vi "报警信息.vi"(11 "报警簇":bool[](array[boolean])) -> (2 "系统报警信息":string, 3 "采配水报警信息":string)   [LabVIEW 2016, in "PLC.lvlib"]
uses:
  PLC.lvlib
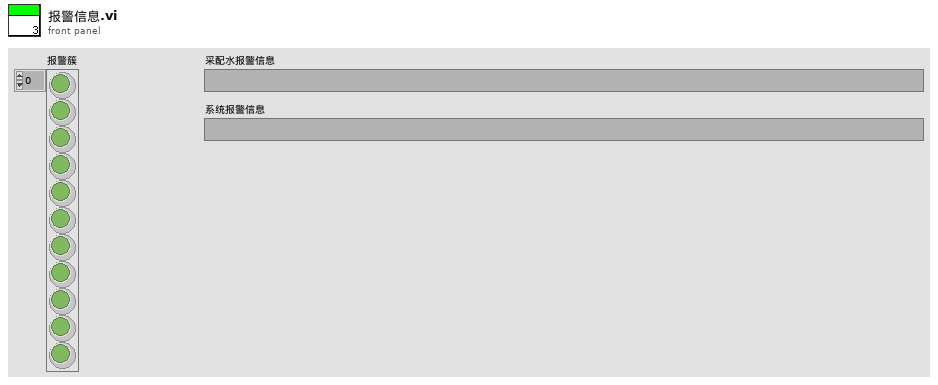
[diagram p1: front panel]
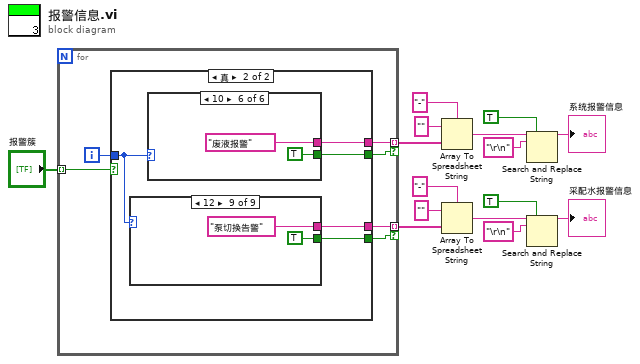
[diagram p0: block diagram]
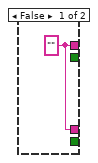
[diagram p2: hidden frame]
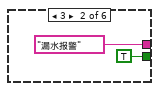
[diagram p4: hidden frame]
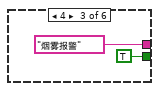
[diagram p5: hidden frame]
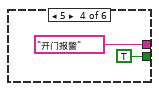
[diagram p6: hidden frame]
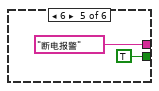
[diagram p7: hidden frame]
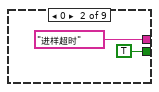
[diagram p9: hidden frame]
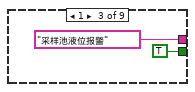
[diagram p10: hidden frame]
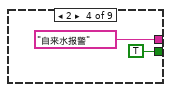
[diagram p11: hidden frame]
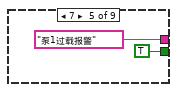
[diagram p12: hidden frame]
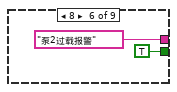
[diagram p13: hidden frame]
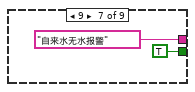
[diagram p14: hidden frame]
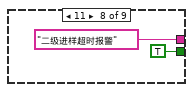
[diagram p15: hidden frame]
diagram:
  n1 = for {
    tunnel: "报警簇" -> [w19] mode=indexing
    tunnel: [w20] -> w2 mode=indexing if=w18
    tunnel: [w17] -> w1 mode=indexing if=w16
    i -> [w21]
    n2 = case shown="真" w19 {
      tunnel: w21 -> [_ w23]
      tunnel: [w22 w27] -> w20
      tunnel: [_ w26] -> w18
      tunnel: [w22 w25] -> w17
      tunnel: [_ w24] -> w16
      frame False {
        w22 = ""
      }
      frame True {
        n3 = case shown="12" w23 {
          tunnel: [_ "进样超时" ("组合框") "采样池液位报警" ("组合框") "自来水报警" ("组合框") "泵1过载报警" ("组合框") "泵2过载报警" ("组合框") "自来水无水报警" ("组合框") "二级进样超时报警" ("组合框") "泵切换告警" ("组合框")] -> w27
          tunnel: [_ TRUE TRUE TRUE TRUE TRUE TRUE TRUE TRUE] -> w26
          frame Default {
          }
          frame 0 {
          }
          frame 1 {
          }
          frame 2 {
          }
          frame 7 {
          }
          frame 8 {
          }
          frame 9 {
          }
          frame 11 {
          }
          frame 12 {
          }
        }
        n4 = case shown="10" w23 {
          tunnel: [_ "漏水报警" ("组合框") "烟雾报警" ("组合框") "开门报警" ("组合框") "断电报警" ("组合框") "废液报警" ("组合框")] -> w25
          tunnel: [_ TRUE TRUE TRUE TRUE TRUE] -> w24
          frame Default {
          }
          frame 3 {
          }
          frame 4 {
          }
          frame 5 {
          }
          frame 6 {
          }
          frame 10 {
          }
        }
      }
    }
  }
  n5 = Array To Spreadsheet String(delimiter (Tab)="-" ("分隔符(Tab)"), array=w1, 3:"" ("格式字符串")) -> (spreadsheet string=w11:string)
  n6 = Array To Spreadsheet String(delimiter (Tab)="-" ("分隔符(Tab)"), array=w2, 3:"" ("格式字符串")) -> (spreadsheet string=w5:string)
  n7 = Search and Replace String(replace all?=TRUE ("替换全部？(F)"), input string=w11, search string="\r\n" ("搜索字符串")) -> (result string=→"系统报警信息":string)  [unwired: 5 in, 3 out]
  n8 = Search and Replace String(replace all?=TRUE ("替换全部？(F)"), input string=w5, search string="\r\n" ("搜索字符串")) -> (result string=→"采配水报警信息":string)  [unwired: 5 in, 3 out]
